vi "SQL插入命令.vi"(8 "时间戳":string, 9 "插入数值":string[](array[string]), 10 "段名":string[](array[string]), 11 "table":string) -> (3 "SQL插入命令":string)   [LabVIEW 2016]
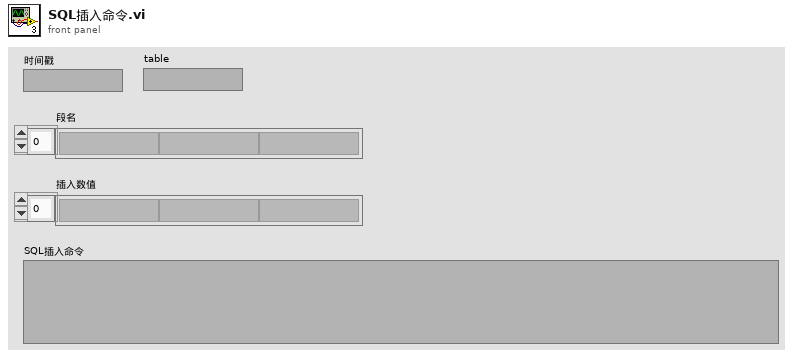
[diagram p1: front panel]
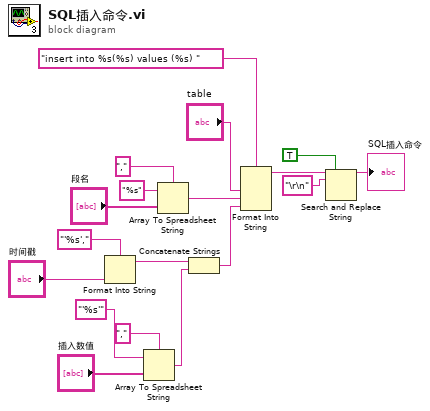
[diagram p0: block diagram]
diagram:
  n1 = Format Into String(format string="'%s'," ("格式字符串"), "时间戳") -> (resulting string=w2:string)  [unwired: 2 in, 1 out]
  n2 = Array To Spreadsheet String(delimiter (Tab)="," ("分隔符(Tab)"), array="插入数值", 3:"'%s'" ("格式字符串")) -> (spreadsheet string=w5:string)
  n3 = Array To Spreadsheet String(delimiter (Tab)="," ("分隔符(Tab)"), array="段名", 3:"%s" ("格式字符串")) -> (spreadsheet string=w10:string)
  n4 = Concatenate Strings(w2, w5) -> (w4:string)
  n5 = Format Into String(format string="insert into %s(%s) values (%s) " ("格式字符串"), "table", w10, w4) -> (resulting string=w14:string)  [unwired: 2 in, 1 out]
  n6 = Search and Replace String(replace all?=TRUE ("替换全部？(F)"), input string=w14, search string="\r\n" ("搜索字符串")) -> (result string=→"SQL插入命令":string)  [unwired: 5 in, 3 out]
